vi "Get Ref Clock Source.vi"(8 "error in (no error)":errorcluster, 11 "VISA resource name":refnum<visa-resource-name>) -> (0 "error out":errorcluster, 2 "Reference Source":u16, 3 "VISA resource name out":refnum<visa-resource-name>)   [LabVIEW 2014, in "Fluke 5XXX Series Multicalibrators.lvlib"]
doc: "This VI returns the reference clock source (internal or through the 10 MHz IN BNC connector).\n\nNote:\n\nThis VI is available only for instrument model 5520A."
uses:
  Fluke 5XXX Series Multicalibrators.lvlib
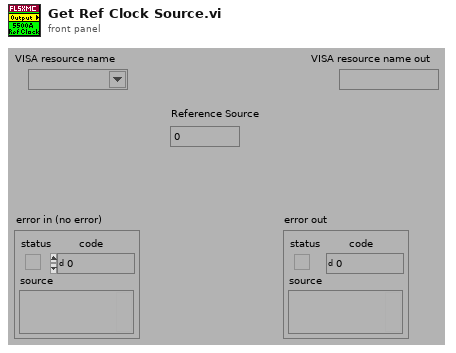
[diagram p1: front panel]
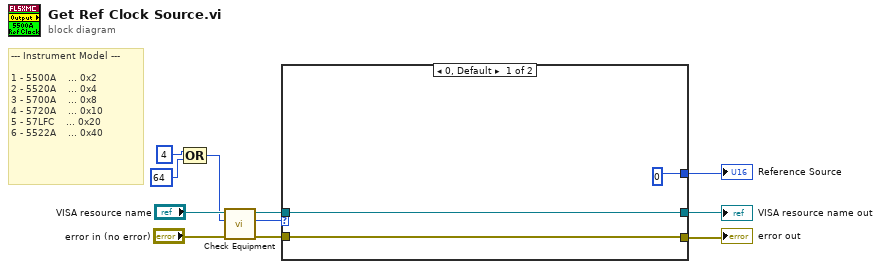
[diagram p0: block diagram]
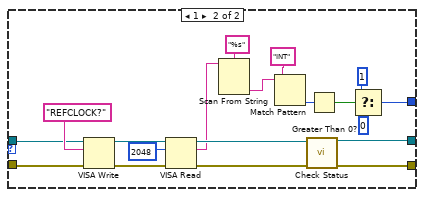
[diagram p2: hidden frame]
diagram:
  # "--- Instrument Model ---\n\n1 - 5500A    ... 0x2\n2 - 5520A    ... 0x4\n3 - 5700A    ... 0x8\n4 - 5720A    ... 0x10\n5 - 57LFC    ... 0x20\n6 - 5522A    ... 0x40"
  n1 = Compound Arithmetic op=OR(4 ("Numeric"), 64 ("Numeric")) -> (w1:i32)
  n2 = call "Check Equipment.vi"("error in (no error)"="error in (no error)", "Bit Mask"=w1, "VISA resource name"="VISA resource name") -> ("error out"=w11:errorcluster, "Present?"=w10:u32, "VISA resource name out"=w9:refnum<visa-resource-name>)  [unwired: 6 in]
  n3 = case shown="0, Default" w10 {
    tunnel: [w13 w27] -> w6
    tunnel: [w12 w24] -> w7
    tunnel: w11 -> [w13 w29]
    tunnel: w9 -> [w12 w28]
    tunnel: [u16 0 w15] -> w8
    frame 0, Default {
    }
    frame 1 {
      n4 = VISA Write(VISA resource name=w28, write buffer="REFCLOCK?", error in (no error)=w29) -> (VISA resource name out=w32:refnum<visa-resource-name>, error out=w31:errorcluster)  [unwired: 1 out]
      n5 = VISA Read(VISA resource name=w32, byte count=u32 2048 ("byte count (0)"), error in (no error)=w31) -> (VISA resource name out=w25:refnum<visa-resource-name>, read buffer=w17:string, error out=w26:errorcluster)  [unwired: 1 out]
      n6 = Scan From String(format string="%s", input string=w17) -> (output 1=w16:string)  [unwired: 3 in, 3 out]
      n7 = Match Pattern(string=w16, regular expression="INT") -> (offset past match=w21:i32)  [unwired: 1 in, 3 out]
      n8 = call "Check Status.vi"("VISA resource name"=w25, "error in (no error)"=w26) -> ("VISA resource name out"=w24:refnum<visa-resource-name>, "error out"=w27:errorcluster)  [unwired: 12 in]
      n9 = Greater Than 0?(x=w21) -> (x > 0?=w18:bool)
      n10 = Select(t=u16 1 ("f"), s=w18, f=u16 0) -> (s? t:f=w15:u16)
    }
  }
  "Reference Source" <- w8
  "VISA resource name out" <- w7
  "error out" <- w6
